vi "SR830 query time constant.vi"(8 "error in (no error)":errorcluster, 11 "VISA resource name":refnum<visa-resource-name>) -> (0 "error out":errorcluster, 2 "time constant":dbl[unit], 3 "VISA resource name out":refnum<visa-resource-name>)   [LabVIEW 2009, in "SR830.lvlib"]
doc: "Reads the current time constant of the lock-in amplifier."
uses:
  sr830/SR830.lvlib
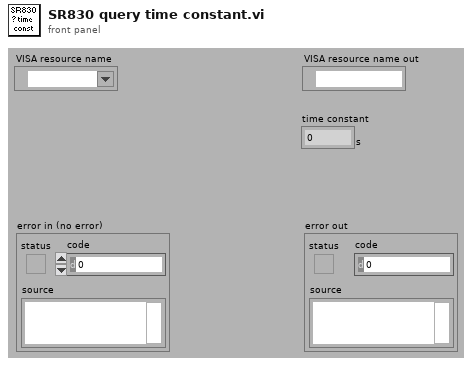
[diagram p1: front panel]
types:
  T1 = typedef "Semaphore RefNum" = refnum<k1>
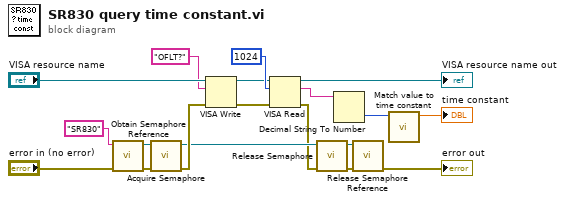
[diagram p0: block diagram]
diagram:
  n1 = call <vilib>:"Obtain Semaphore Reference.vi"("error in (no error)"="error in (no error)", "name (unnamed)"="SR830") -> ("error out"=w13:errorcluster, "semaphore"=w12:T1)  [unwired: 1 in, 3 out]
  n2 = call <vilib>:"Acquire Semaphore.vi"("error in (no error)"=w13, "semaphore"=w12) -> ("error out"=w9:errorcluster, "semaphore out"=w6:T1)  [unwired: 1 in, 3 out]
  n3 = VISA Write(VISA resource name="VISA resource name", write buffer="OFLT?", error in (no error)=w9) -> (VISA resource name out=w18:refnum<visa-resource-name>, error out=w17:errorcluster)  [unwired: 1 out]
  n4 = VISA Read(VISA resource name=w18, byte count=u32 1024 ("bytes to read (1000)"), error in (no error)=w17) -> (VISA resource name out=→"VISA resource name out":refnum<visa-resource-name>, read buffer=w3:string, error out=w5:errorcluster)  [unwired: 1 out]
  n5 = call <vilib>:"Release Semaphore.vi"("error in (no error)"=w5, "semaphore"=w6) -> ("error out"=w8:errorcluster, "semaphore out"=w7:T1)  [unwired: 4 out]
  n6 = Decimal String To Number(string=w3) -> (number=w1:i32)  [unwired: 3 out]
  n7 = call <vilib>:"Release Semaphore Reference.vi"("error in (no error)"=w8, "semaphore"=w7) -> ("error out"=→"error out":errorcluster)  [unwired: 9 out]
  n8 = call "Match value to time constant.vi"("integer"=w1) -> ("time constant"=→"time constant":dbl[unit])  [unwired: 10 out]
